vi "Document_GetCommonStyles.vi"(8 "error in":errorcluster, 11 "Document in":refnum<k24>) -> (0 "error out":errorcluster, 2 "Common Styles":string[](array[string]), 3 "Document out":refnum<k24>)   [LabVIEW 2009]
uses:
  C:/Users/François/Documents/Programmation/_ooReport/DLLs/AODL.dll
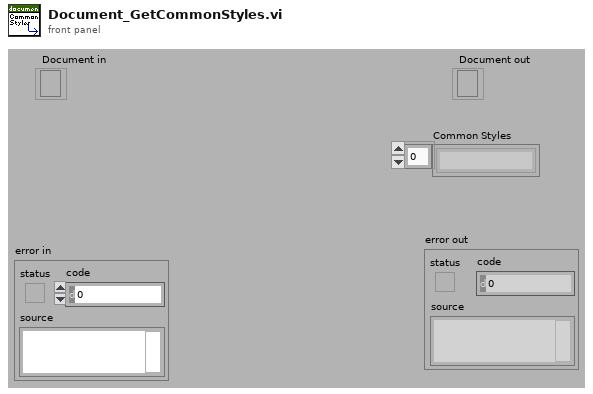
[diagram p1: front panel]
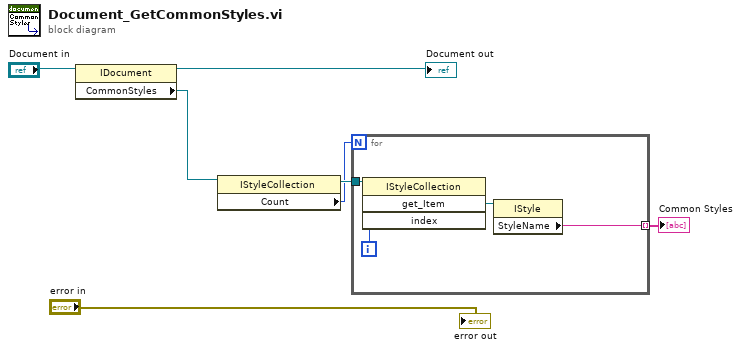
[diagram p0: block diagram]
diagram:
  n1 = property class="IDocument"(reference="Document in") -> (reference out=→"Document out":refnum<k24>, "CommonStyles"=w5:refnum<k24>)  [unwired: 1 in, 1 out]
  n2 = property class="IStyleCollection"(reference=w5) -> (reference out=w4:refnum<k24>, "Count"=w3:i32)  [unwired: 1 in, 1 out]
  n3 = for {
    N: w3 -> [_]
    tunnel: w4 -> [w11]
    tunnel: [w8] -> w2 mode=indexing
    i -> [w10]
    n4 = invoke class="IStyleCollection" method="get_Item"(reference=w11, "index"=w10) -> ("get_Item"=w9:refnum<k24>)  [unwired: 2 in, 3 out]
    n5 = property class="IStyle"(reference=w9) -> ("StyleName"=w8:string)  [unwired: 1 in, 2 out]
  }
  "Common Styles" <- w2
  "error out" <- "error in"
